vi "gate sts with current adjustment.vi"() -> ()   [LabVIEW 2010]
uses:
  <vilib>/Utility/file.llb/Read From Spreadsheet File (DBL).vi
  <userlib>/Nanonis Prog Interface V5/Nanonis Prog Interface.lvlib
panel:
  in  "Notes":string
  in  "Minimum Current":dbl=1e-11
  in  "Starting Index":i32=1
  in  "File with Current Data":string
  out "Index":i32
  out "Current Gate Voltage (V)":dbl
  in  "Stop":bool
  in  "Basename":string
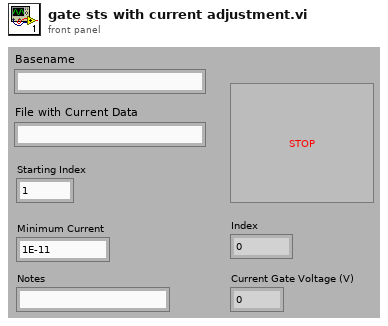
[diagram p1: front panel]
types:
  T1 = cluster{"Save all":enum16{"no change", "on", "off"}, "Number of Sweeps (0=no change)":i32}
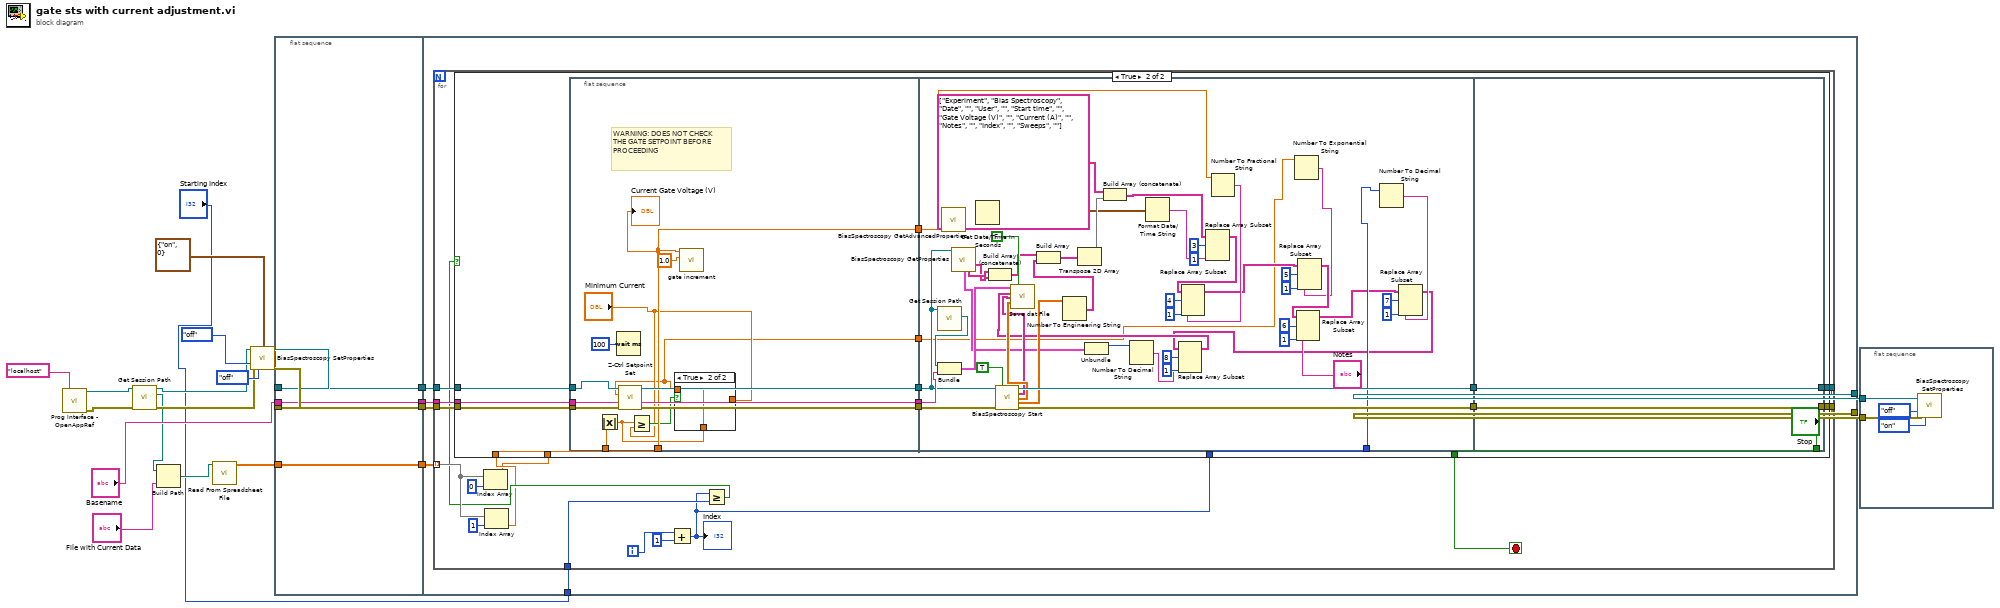
[diagram p0: block diagram]
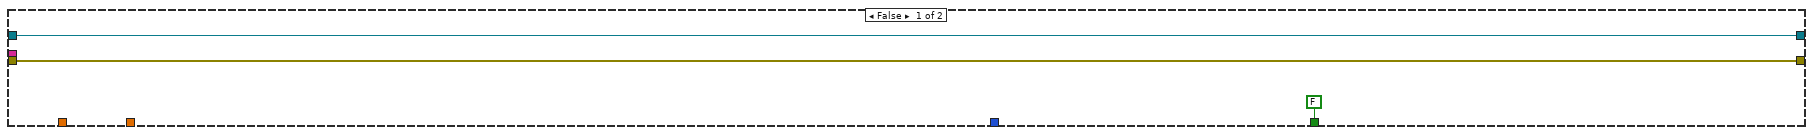
[diagram p2: hidden frame]
diagram:
  n1 = call <userlib>:"Prog Interface - OpenAppRef.vi"("Machine name (local machine IP)"="localhost" ("machine name (localhost)")) -> ("Error out"=w10:errorcluster, "Application reference"=w7:refnum<vi>)  [unwired: 5 in]
  n2 = call <userlib>:"Get Session Path.vi"("error in (no error)"=w10, "Application ref in"=w7) -> ("error out"=w9:errorcluster, "Session path"=w6:path, "Application ref out"=w8:refnum<vi>)  [unwired: 7 in]
  n3 = Build Path(base path=w6, name or relative path="File with Current Data") -> (appended path=w4:path)
  n4 = call-poly <vilib>:"Read From Spreadsheet File.vi"("file path (dialog if empty)"=w4) -> ("all rows"=w3:dbl[][])  [unwired: 6 in, 4 out]
  n5 = call <userlib>:"BiasSpectroscopy SetProperties.vi"("Application ref in"=w8, "Autosave (no change)"=enum16{"no change", "on", "off"}."off", "Error in (no error)"=w9, "Save dialog"=enum16{"no change", "on", "off"}."off", "Multiple sweeps config"=T1 {"Save all"=enum."on", "Number of Sweeps (0=no change)"=0}) -> ("Application ref out"=w19:refnum<vi>, "Error out"=w20:errorcluster)  [unwired: 9 in]
  n6 = flat-sequence {
    tunnel: w19 -> [w24]
    tunnel: w20 -> [w25]
    tunnel: "Basename" -> [w26]
    tunnel: [w26] -> w14
    tunnel: [w25] -> w13
    tunnel: [w24] -> w12
    tunnel: w3 -> [w23]
    tunnel: [w23] -> w2
    tunnel: [w30] -> w17
    tunnel: [w29] -> w16
    tunnel: w14 -> [w33]
    tunnel: w13 -> [w32]
    tunnel: w12 -> [w31]
    tunnel: w2 -> [w28]
    tunnel: "Starting Index" -> [w27]
    frame #0 {
    }
    frame #1 {
      n7 = for {
        tunnel: w33 -> [w49]
        tunnel: w32 -> [w48]
        tunnel: w31 -> [w47]
        tunnel: [w46] -> w30
        tunnel: [w45] -> w29
        tunnel: w28 -> [w41] mode=indexing
        tunnel: w27 -> [w38]
        i -> [w43]
        stop <- w44 stop-if-true
        n8 = Index Array(array=w41, index=0) -> (element=w35:dbl)
        n9 = Index Array(array=w41, index=1) -> (element=w36:dbl)
        n10 = Add(x=w43, y=1) -> (x+y=w34:i32)
        "Index" <- w34
        n11 = Greater Or Equal?(x=w34, y=w38) -> (x >= y?=w37:bool)
        n12 = case shown="True" w37 {
          tunnel: w49 -> [_ w63]
          tunnel: w48 -> [w51 w62]
          tunnel: w47 -> [w52 w61]
          tunnel: [w52 w60] -> w46
          tunnel: [w51 w59] -> w45
          tunnel: [FALSE ("Stop") w58] -> w44
          tunnel: w36 -> [_ w57]
          tunnel: w35 -> [_ w56]
          tunnel: w34 -> [_ w53]
          frame False {
          }
          frame True {
            n13 = flat-sequence {
              tunnel: w61 -> [w79]
              tunnel: w62 -> [w77]
              tunnel: w63 -> [w81]
              tunnel: [w81] -> w68
              tunnel: [w76] -> w67
              tunnel: [w78] -> w66
              tunnel: w57 -> [w75]
              tunnel: w56 -> [w73]
              tunnel: [w73] -> w55
              tunnel: [w69] -> w54
              tunnel: [w131] -> w65
              tunnel: [w132] -> w64
              tunnel: w68 -> [w124]
              tunnel: w67 -> [w133]
              tunnel: w66 -> [w123]
              tunnel: w55 -> [w99]
              tunnel: w54 -> [w90]
              tunnel: w53 -> [w89]
              tunnel: [w135] -> w60
              tunnel: [w136] -> w59
              tunnel: ["Stop"] -> w58
              tunnel: w64 -> [w135]
              tunnel: w65 -> [w136]
              frame #0 {
                # "WARNING: DOES NOT CHECK THE GATE SETPOINT BEFORE PROCEEDING"
                n14 = Absolute Value(x=w75) -> (abs(x)=w71:dbl)
                n15 = Wait (ms)(milliseconds to wait=u32 100) -> ()  [unwired: 1 out]
                n16 = Greater Or Equal?(x=w71, y="Minimum Current") -> (x >= y?=w72:bool)
                n17 = case shown="True" w72 {
                  tunnel: w71 -> [_ w83]
                  tunnel: [w82 w83] -> w69
                  tunnel: "Minimum Current" -> [w82 _]
                  frame False {
                  }
                  frame True {
                  }
                }
                n18 = call <userlib>:"Z-Ctrl Setpoint Set.vi"("error in (no error)"=w77, "Z Controller setpoint"=w69, "Application ref in"=w79) -> ("error out"=w76:errorcluster, "Application ref out"=w78:refnum<vi>)  [unwired: 7 in]
                n19 = call "gate increment.vi"("Increment"=1.0, "Gate Voltage"=w73) -> ()  [unwired: 10 in]
                "Current Gate Voltage (V)" <- w73
              }
              frame #1 {
                n20 = call <userlib>:"Get Session Path.vi"("Application ref in"=w123) -> ("Session path"=w129:path)  [unwired: 8 in, 2 out]
                n21 = Bundle("Session path"=w129, "Basename"=w124) -> (w128:cluster{"Session path":path, "Basename":string})  [unwired: 1 in]
                n22 = call <userlib>:"BiasSpectroscopy GetAdvancedProperties.vi"() -> ()  [unwired: 10 in, 6 out]
                n23 = call <userlib>:"BiasSpectroscopy GetProperties.vi"("Application ref in"=w123) -> ("Parameters"=w115:string[], "Multiple sweeps configuration"=w105:cluster{"Number of Sweeps":i32, "Save all":bool}, "Fixed parameters"=w116:string[])  [unwired: 7 in, 5 out]
                n24 = Get Date/Time In Seconds() -> (seconds since 1Jan1904=w114:timestamp)
                n25 = Build Array (concatenate)(w116, w115) -> (w120:string[])
                n26 = call <userlib>:"BiasSpectroscopy Start.vi"("Application ref in"=w123, "Get data (F)"=TRUE, "Error in (no error)"=w133) -> ("Application ref out"=w132:refnum<vi>, "Channels"=w126:string[], "Data"=w127:sgl[][], "Parameters"=w122:sgl[], "Error out"=w131:errorcluster)  [unwired: 8 in]
                n27 = Number To Engineering String(4:w122) -> (0:w121:string[])  [unwired: 3 in]
                n28 = Build Array(w120, w121) -> (w119:string[][])
                n29 = Transpose 2D Array(2D array=w119) -> (transposed array=w117:string[][])
                n30 = Unbundle(w105) -> ("Number of Sweeps"=w104:i32)  [unwired: 1 out]
                n31 = Build Array (concatenate)(string[][] [["Experiment", "Bias Spectroscopy"], ["Date", ""], ["User", ""], ["Start time", ""], ["Gate Voltage (V)", ""], ["Current (A)", ""], ["Notes", ""], ["Index", ""], ["Sweeps", ""]] ("Attributes"), w117) -> (w113:string[][])
                n32 = Number To Decimal String(number=w104) -> (decimal integer string=w100:string)  [unwired: 1 in]
                n33 = Format Date/Time String(seconds (now)=w114) -> (date/time string=w112:string)  [unwired: 2 in]
                n34 = Replace Array Subset(array=w113, new element=w112, index (row)=3, index (col)=1 ("disabled index (col)")) -> (w109:string[][])
                n35 = Number To Fractional String(number=w99) -> (F-format string=w106:string)  [unwired: 3 in]
                n36 = Replace Array Subset(array=w109, new element=w106, index (row)=4, index (col)=1 ("disabled index (col)")) -> (w93:string[][])
                n37 = Number To Exponential String(number=w90) -> (E-format string=w91:string)  [unwired: 3 in]
                n38 = Replace Array Subset(array=w93, new element=w91, index (row)=5, index (col)=1 ("disabled index (col)")) -> (w94:string[][])
                n39 = Replace Array Subset(array=w94, new element="Notes", index (row)=6, index (col)=1 ("disabled index (col)")) -> (w85:string[][])
                n40 = Number To Decimal String(number=w89) -> (decimal integer string=w86:string)  [unwired: 1 in]
                n41 = Replace Array Subset(array=w85, new element=w86, index (row)=7, index (col)=1 ("disabled index (col)")) -> (w84:string[][])
                n42 = Replace Array Subset(array=w84, new element=w100, index (row)=8, index (col)=1 ("disabled index (col)")) -> (w103:string[][])
                n43 = call <userlib>:"Save dat File.vi"("Filename control"=w128, "Show save dialog (T)"=FALSE, "Attributes"=w103, "Channels names"=w126, "Data"=w127) -> ()  [unwired: 7 in, 4 out]
              }
              frame #2 {
              }
            }
          }
        }
      }
    }
  }
  n44 = flat-sequence {
    tunnel: w17 -> [w140]
    tunnel: w16 -> [w139]
    frame #0 {
      n45 = call <userlib>:"BiasSpectroscopy SetProperties.vi"("Application ref in"=w140, "Autosave (no change)"=enum16{"no change", "on", "off"}."off", "Error in (no error)"=w139, "Save dialog"=enum16{"no change", "on", "off"}."on") -> ()  [unwired: 10 in, 2 out]
    }
  }
